vi "New.vi"(7 "Entity Manager":refnum<class "Entity Manager.lvclass">, 11 "Entity in":refnum<class "Entity.lvclass">) -> (3 "Entity out":refnum<class "Entity.lvclass">)   [LabVIEW 2020, in "Conditum.lvlib" / "Entity.lvclass"]
uses:
  Entity.lvclass
  Entity State.ctl
  Entity.lvclass/Entity.ctl
  Columns/ID/ID.lvclass
  Conditum.lvlib
  Entity Manager/Entity Manager.lvclass
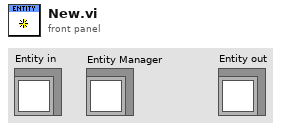
[diagram p1: front panel]
types:
  T1 = typedef "Conditum.lvlib/Entity State.ctl" = enum16{"New", "Managed", "Detached", "Removed"}
  T2 = typedef "Conditum.lvlib/Entity ID.ctl" = i64
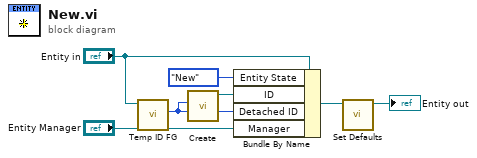
[diagram p0: block diagram]
diagram:
  n1 = call "Temp ID FG.vi"("Entity"="Entity in") -> ("New ID"=w4:T2)  [unwired: 10 in]
  n2 = call "Create.vi"("Entity ID"=w4) -> ("ID out"=w6:refnum<class "ID.lvclass">)  [unwired: 10 in]
  n3 = Bundle By Name(cluster="Entity in", "Entity State"=Entity_State."New", "ID"=w6, "Detached ID"=w4, "Manager"="Entity Manager") -> (w3:refnum<class "Entity.lvclass">)
  n4 = call-dynamic "Set Defaults.vi"("Entity in"=w3) -> ("Entity out"=→"Entity out":refnum<class "Entity.lvclass">)  [unwired: 10 in]
